vi "Lidar Master V5.2.vi"() -> ()   [LabVIEW 2015]
uses:
  Controls/FPGA Nain State.ctl
  <vilib>/Platform/TimedLoop/XDataNode/timing_clust.ctl
  <vilib>/Platform/TimedLoop/XDataNode/nitl_modes.ctl
  <vilib>/Platform/TimedLoop/XDataNode/wakeup.ctl
  <vilib>/rvi/Emulation/niFpgaGetClockAttributes.vi
  <vilib>/rvi/Emulation/niFpgaSctlEmulationGetInTimedLoop.vi
  <vilib>/rvi/Emulation/niFpgaEmulationReportErrorSimple.vi
  <vilib>/rvi/eio/common/nirviEmuTemplateMethod_errors.vi
  <vilib>/rvi/Emulation/niFpgaCriticalErrorInLSC.vi
  <vilib>/rvi/Emulation/niFpgaProcessEmulError.vi
  <vilib>/rvi/Memory/Memory_Emulation/nirvimemoryFastEmulation.vi
  <vilib>/rvi/Memory/Memory_Emulation/nirvimemoryEmulation.vi
  <vilib>/rvi/Emulation/niFpgaEmulationIsFPGAContextNoSignature.vi
  <vilib>/rvi/DataTransferAndStorage/Container/Common/niFpgaContainerGetUniqueNameForEmu.vi
  <vilib>/rvi/errors/nirviReportUnexpectedCaseInternalError (U32).vi
  <vilib>/rvi/errors/niFpgaSetErrorForExecOnDevCompSimple.vi
  <vilib>/rvi/eio/common/nirviEmuReportErrorAndStop.vi
  <vilib>/rvi/FIFO/Fifo_Resource/nirvififoEmulationSetSize.vi
  <vilib>/rvi/FIFO/Fifo_Resource/nirviFifoEmulationQueueMgr.vi
  <instcachedir>/0/nirviFifoEmulationQueueMgr_E5CAEC123FF24DC58D834DCA3CDAA9B5.lvgen/nirviFifoEmulationQueueMgr_E5CAEC123FF24DC58D834DCA3CDAA9B5_002.vi
  <vilib>/Utility/error.llb/Clear Errors.vi
  <vilib>/rvi/FIFO/Fifo_Resource/nirvififoEmulationCreateLock.vi
  <vilib>/rvi/FIFO/Fifo_Resource/nirvififoEmulationObtainLock.vi
  <vilib>/rvi/FIFO/Fifo_Resource/nirvififoEmulationReleaseLock.vi
  <vilib>/rvi/occurrence/nirviWaitOnOccurrenceBase.vi
  <vilib>/rvi/errors/nirviReportUnexpectedCaseInternalError.vi
  <vilib>/eio/EIONode/EIONode.xnode
  <vilib>/Platform/TimedLoop/XDataNode/XDataNode.xnode
  <vilib>/rvi/DataTransferAndStorage/Container/XNode/niFpgaContainer.xnode
  <vilib>/rvi/FIFO/Fifo_Resource/nirvififoEmulationRead.vi
  <vilib>/eio/EIOMethodNode/EIOMethodNode.xnode
  <vilib>/Platform/TimedLoop/XDataNode/XDNodeRunTimeDep.lvlib
  LIDAR V2 Globals.vi
panel:
  in  "VgaStart":u8
  in  "User Command Commit":bool
  in  "User Command":u8
  in  "User Data 1":u8
  in  "User Data 0":u8
  in  "StartSyncLoop":bool
  out "Trig1":bool
  in  "SendDebugVal":bool
  in  "WriteSenseData":i16
  in  "WriteSensAdd":i16
  in  "WriteSensDataEn":bool
  in  "ActiveSensDeb":u8
  in  "SensScanDeb":bool
  in  "SensorMap":u8[](array[numeric])=[0, 0, 0, 0, 0, 0, 0, 0, 0, 0, 0, 0, 1, 1, 1, 1, 1, 1, 1, 1, 1, 1, 1, 1, 0, 0, 0, 0, 0, 0, 0, 0, 0, 0, 0, 0, 1, 1, 1, 1, 1, 1, 1, 1, 1, 1, 1, 1, 2, 2, 2, 2, 2, 2, 2, 2, 2, 2, 2, 2, 3, 3, 3, 3, 3, 3, 3, 3, 3, 3, 3, 3, 2, 2, 2, 2, 2, 2, 2, 2, 2, 2, 2, 2, 3, 3, 3, 3, 3, 3, 3, 3, 3, 3, 3, 3]
  in  "AiNoOfSamples":u16=99
  out "User Command Idle":bool
  out "User Command Status":u8
  out "User Error":bool
  out "Configured?":bool
  out "PLL Locked":bool
  in  "SendAiCMD":u16
  in  "NoOfSamples":u16=1247
  in  "DOActivate":u16=10
  in  "PulseEnd":u16=25
  in  "VgaAdd":u32
  in  "VgaData":i16
  in  "FillVga":bool
  in  "PowerBit0":bool
  in  "PowerBit1":bool
  in  "ActiveLedIndexDeb":u16
  in  "LedScanDebEn":bool
  out "Port0":u8=2 format="%.0b"
  out "Port1Bit4":bool
  out "Port1Bit5":bool
  out "Port1":u8 format="%.0b"
  in  "ScanMode":bool
  out "PulseIndex":i16=88
  in  "StartAcq":u16=26
  in  "StartPulse":u16=20
  in  "StartES":u16=15
  in  "StopES":u16=30
  out "EnableSignal":bool
  out "ActiveLedIndex":u16=2
  in  "EndOfPulseGen":bool=TRUE
  in  "SamplingEnable":bool
  in  "SingleFrame":bool
  out "MainState":T1=enum."ActivatePulseCycle"
  in  "NoOfLeds":u16=95
  in  "PulsePerLed":i16=199
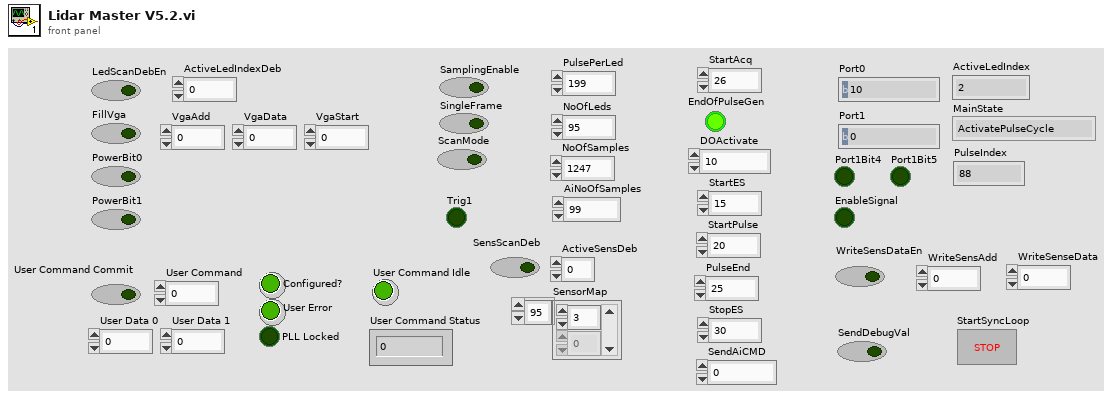
[diagram p1: front panel]
types:
  T1 = typedef "FPGA Nain State.ctl" = enum16{"WaitForStart", "SelectActiveLed", "WaitForNextPulse", "ActivatePulseCycle", "Error"}
  T2 = typedef "XDNodeRunTimeDep.lvlib/timing_clust.ctl" = cluster{"Expected End [f-1]":u64, "Actual End [f-1]":u64, "Finished Late? [f-1]":bool, "Expected End [i-1]":u64, "Actual End [i-1]":u64, "Finished Late? [i-1]":bool, "Expected Start [i]":u64, "Actual Start [i]":u64, "Expected Start [f]":u64, "Actual Start [f]":u64, "Source Name":string, "Structure Name":string, "Period":i64, "Deadline":i64, "Offset":i64, "Start":i64, "Priority":i32, "Timeout":i32, "Mode":T3, "Wakeup Reason":T4, "Error":errorcluster, "Source Type":string, "Secondary Source Type":string, "Global End Time":u64, "Global Start Time":u64, "Frame Duration":u64, "Iteration Duration":u64, "Assigned CPU":i32, "I/O Scan Engine Mode":u32}
  T3 = typedef "XDNodeRunTimeDep.lvlib/nitl_modes.ctl" = enum32{"No Change", "Process missed periods, maintain original phase", "Discard missed periods, maintain original phase", "Process missed periods, ignore original phase", "Discard missed periods, ignore original phase"}
  T4 = typedef "XDNodeRunTimeDep.lvlib/wakeup.ctl" = enum32{"Normal", "Aborted", "Asynchronous wakeup", "Timing source error", "Timed loop error", "Timeout"}
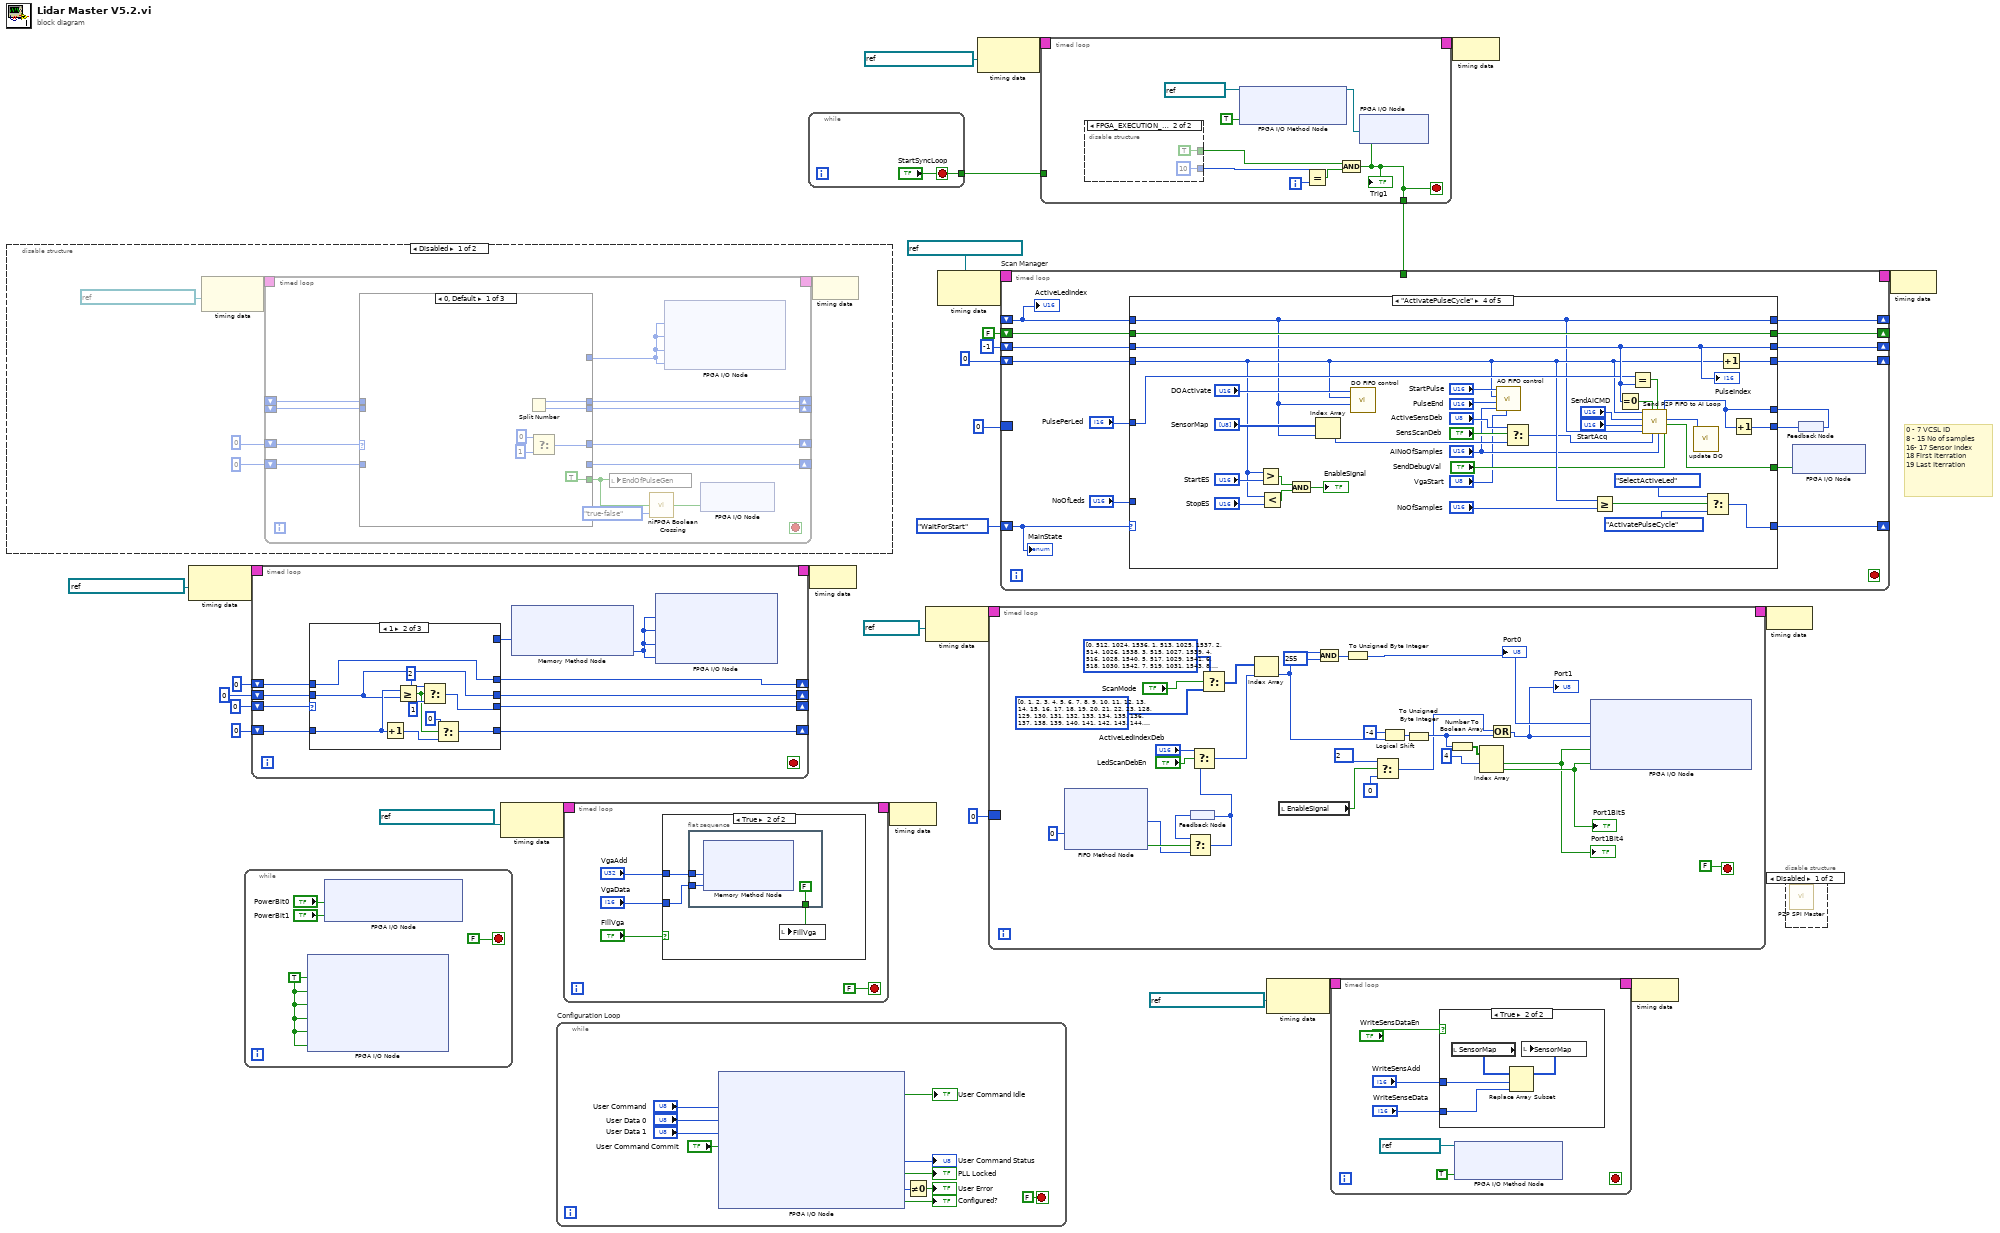
[diagram p0: block diagram]
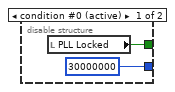
[diagram p3: hidden frame]
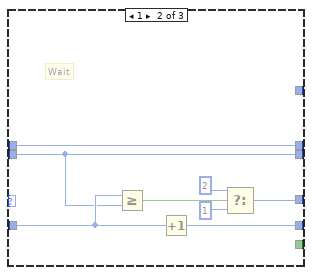
[diagram p5: hidden frame]
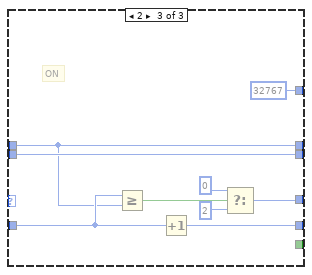
[diagram p6: hidden frame]
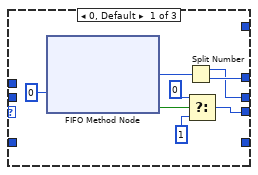
[diagram p8: hidden frame]
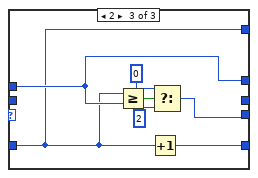
[diagram p9: hidden frame]
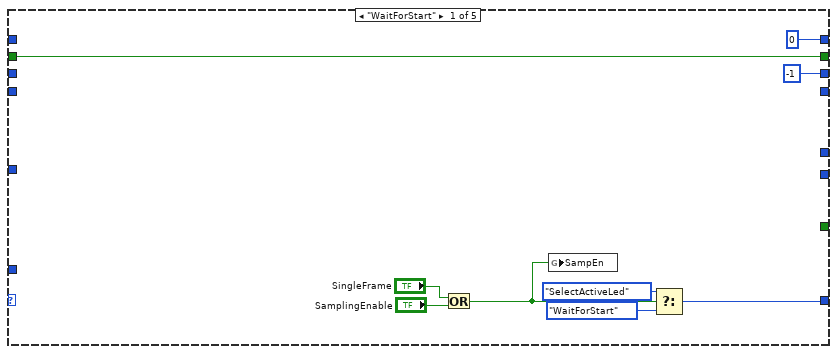
[diagram p11: hidden frame]
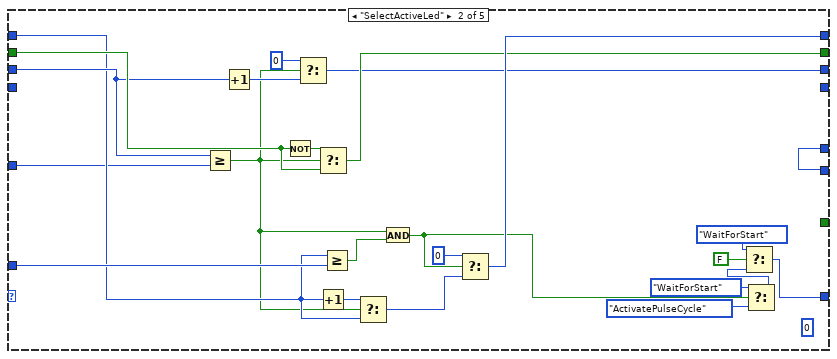
[diagram p12: hidden frame]
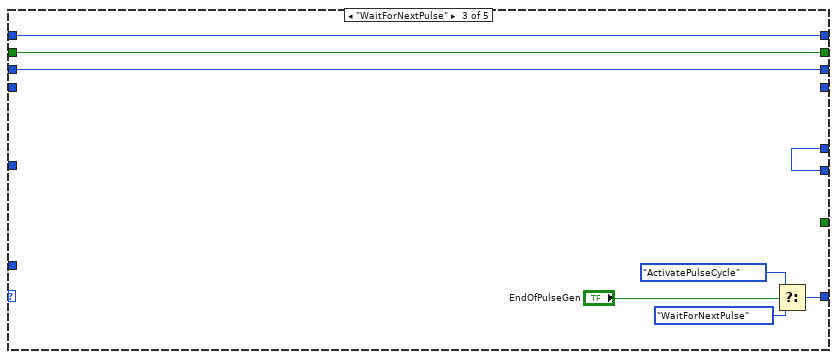
[diagram p13: hidden frame]
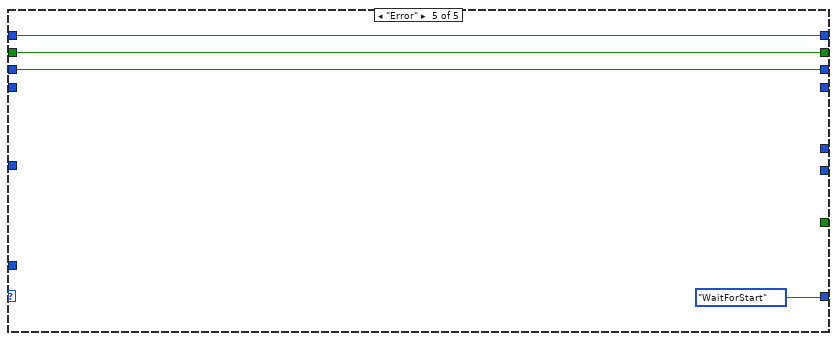
[diagram p14: hidden frame]
diagram:
  # "0 - 7 VCSL ID\n8 - 15 No of samples\n16- 17 Sensor index\n18 First Iterration\n19 Last Iterration"
  n1 = disable-structure shown="Disabled" {
    frame Disabled {
      n2 = node-c288(refnum<k21> "IO Module\\Data Clock" ("Source Name")) -> (w35:T2)
      n3 = timed-loop {
        timing: w35 -> [_]
        timing-out: [_] -> w34
        shift-right: [w46] -> _
        shift-left: i16 0 -> [w47]
        shift-right: [w45] -> _
        shift-left: u32 0 -> [w39]
        shift-right: [w44] -> _
        shift-left: _ -> [w42]
        shift-right: [w43] -> _
        shift-left: _ -> [w41]
        stop <- _ stop-if-true
        n4 = case shown="0, Default" w47 {
          tunnel: [w52 w60 w69] -> w46
          tunnel: [_ w62 w71] -> w45
          tunnel: w39 -> [_ w61 w70]
          tunnel: [w50 w58 w67] -> w44
          tunnel: [w49 w55 w64] -> w43
          tunnel: w42 -> [_ w58 w67]
          tunnel: w41 -> [_ w55 w64]
          tunnel: [_ _ i16 32767 ("IO Module\\AO 0 N")] -> w40
          tunnel: [TRUE _ _] -> w38
          frame 0, Default {
            n5 = Split Number() -> (hi(x)=w49:u16, lo(x)=w50:u16)  [unwired: 1 in]
            n6 = Select(t=i16 0, f=i16 1) -> (s=w54:bool, s? t:f=w52:i16)
          }
          frame 1 {
            # "Wait"
            n7 = Greater Or Equal?(x=w61, y=w58) -> (x >= y?=w59:bool)
            n8 = Increment(x=w61) -> (x+1=w62:u32)
            n9 = Select(t=i16 2, s=w59, f=i16 1) -> (s? t:f=w60:i16)
          }
          frame 2 {
            # "ON"
            n10 = Greater Or Equal?(x=w70, y=w64) -> (x >= y?=w68:bool)
            n11 = Increment(x=w70) -> (x+1=w71:u32)
            n12 = Select(t=i16 0, s=w68, f=i16 2) -> (s? t:f=w69:i16)
          }
        }
        n13 = local write "EndOfPulseGen"(w38) -> ()
        n14 = call <vilib>:"niFPGA Boolean Crossing.vi"("input"=w38, "direction"=enum8{"either", "false-true", "true-false"}."true-false") -> ("crossing"=w36:bool)  [unwired: 7 in]
        n15 = xnode "FPGA I/O Node"("IO Module\\AO 0 N-3"=w40, "IO Module\\AO 0 N-2"=w40, "IO Module\\AO 0 N-1"=w40, "IO Module\\AO 0 N"=w40) -> ()  [unwired: 4 in, 4 out]
        n16 = xnode "FPGA I/O Node"("PXI_Trig0"=w36) -> ()  [unwired: 1 in, 1 out]
      }
      n17 = node-c288(w34) -> ()
    }
    frame Enabled {
    }
  }
  n18 = node-c288(refnum<k21> "IO Module\\Data Clock" ("Source Name")) -> (w17:T2)
  n19 = while {
    stop <- FALSE stop-if-true
    w78 = TRUE ("IO Module\\PFI 0 WE")
    n20 = xnode "FPGA I/O Node"("IO Module\\PFI 0 WE"=w78, "IO Module\\PFI 1 WE"=w78, "IO Module\\PFI 2 WE"=w78, "IO Module\\PFI 3 WE"=w78, "IO Module\\DIO Port 0 WE"=w78, "IO Module\\DIO Port 1 WE"=w78) -> ()  [unwired: 6 in, 6 out]
    n21 = xnode "FPGA I/O Node"("IO Module\\PFI 2 Wr Data"="PowerBit0", "IO Module\\PFI 3 Wr Data"="PowerBit1") -> ()  [unwired: 2 in, 2 out]
  }
  n22 = timed-loop {
    timing: w17 -> [_]
    timing-out: [_] -> w16
    shift-right: [w88] -> _
    shift-left: u16 0 -> [w87]
    shift-right: [w89] -> _
    shift-left: u8 0 -> [w90]
    shift-right: [w86] -> _
    shift-left: u16 0 ("Element") -> [w85]
    shift-right: [w84] -> _
    shift-left: u8 0 -> [w83]
    stop <- _ stop-if-true
    n23 = case shown="1" w90 {
      tunnel: [w95 w104 w112] -> w89
      tunnel: w87 -> [_ w109 w110]
      tunnel: [_ w102 w116] -> w88
      tunnel: w85 -> [_ w106 w111]
      tunnel: [w93 w106 w111] -> w86
      tunnel: [w92 w105 _] -> w84
      tunnel: w83 -> [_ w105 _]
      tunnel: [_ _ w110] -> w82
      frame 0, Default {
        n24 = xnode ("FIFO Method Node")("Timeout"=0) -> ("Element"=w94:u16, "Timed Out?"=w98:bool)  [unwired: 1 in, 1 out]
        n25 = Split Number(x=w94) -> (hi(x)=w92:u8, lo(x)=w93:u8)
        n26 = Select(t=u8 0, s=w98, f=u8 1) -> (s? t:f=w95:u8)
      }
      frame 1 {
        n27 = Increment(x=w109) -> (x+1=w103:u16)
        n28 = Greater Or Equal?(x=w109, y=w105) -> (x >= y?=w100:bool)
        n29 = Select(t=u8 2, s=w100, f=u8 1) -> (s? t:f=w104:u8)
        n30 = Select(t=u16 0, s=w100, f=w103) -> (s? t:f=w102:u16)
      }
      frame 2 {
        n31 = Greater Or Equal?(x=w110, y=w111) -> (x >= y?=w115:bool)
        n32 = Increment(x=w110) -> (x+1=w116:u16)
        n33 = Select(t=u8 0, s=w115, f=u8 2) -> (s? t:f=w112:u8)
      }
    }
    n34 = xnode ("Memory Method Node")("Address"=w82) -> ("Data"=w91:i16)  [unwired: 1 in, 1 out]
    n35 = xnode "FPGA I/O Node"("IO Module\\AO 1 N-3"=w91, "IO Module\\AO 1 N-2"=w91, "IO Module\\AO 1 N-1"=w91, "IO Module\\AO 1 N"=w91) -> ()  [unwired: 4 in, 4 out]
  }
  n36 = node-c288(refnum<k21> "IO Module\\Data Clock" ("Source Name")) -> (w21:T2)
  n37 = while "Configuration Loop" {
    stop <- FALSE stop-if-true
    n38 = xnode "FPGA I/O Node"("IO Module\\User Command"="User Command", "IO Module\\User Data 0"="User Data 0", "IO Module\\User Data 1"="User Data 1", "IO Module\\User Command Commit"="User Command Commit") -> ("IO Module\\User Command Idle"=→"User Command Idle":bool, "IO Module\\User Command Status"=→"User Command Status":u8, "IO Module\\PLL Locked"=→"PLL Locked":bool, "IO Module\\User Error"=w126:u8, "IO Module\\Initialization Done"=→"Configured?":bool)  [unwired: 9 in, 9 out]
    n39 = Not Equal To 0?(x=w126) -> (x != 0?=→"User Error":bool)
  }
  n40 = timed-loop {
    timing: w21 -> [_]
    timing-out: [_] -> w20
    stop <- FALSE stop-if-true
    n41 = case shown="True" "FillVga" {
      tunnel: "VgaAdd" -> [_ w136]
      tunnel: "VgaData" -> [_ w135]
      frame False {
      }
      frame True {
        n42 = flat-sequence {
          tunnel: w136 -> [w139]
          tunnel: w135 -> [w138]
          tunnel: [FALSE ("FillVga")] -> w134
          frame #0 {
            n43 = xnode ("Memory Method Node")("Address"=w139, "Data"=w138) -> ()  [unwired: 1 in, 1 out]
          }
        }
        n44 = local write "FillVga"(w134) -> ()
      }
    }
  }
  n45 = while {
    tunnel: ["StartSyncLoop"] -> w2
    stop <- "StartSyncLoop" stop-if-true
  }
  n46 = node-c288(w16) -> ()
  n47 = node-c288(w20) -> ()
  n48 = node-c288(refnum<k21> "130MHz" ("Source Name")) -> (w28:T2)
  n49 = node-c288(refnum<k21> "IO Module\\Data Clock" ("Source Name")) -> (w30:T2)
  n50 = node-c288(refnum<k21> "PXI Clk10 MHz Clock" ("Source Name")) -> (w6:T2)
  n51 = timed-loop {
    timing: w28 -> [_]
    timing-out: [_] -> w27
    border: u16 0 ("Element") -> [_]
    stop <- FALSE stop-if-true
    n52 = xnode ("FIFO Method Node")("Timeout"=0) -> ("Element"=w151:u16, "Timed Out?"=w152:bool)  [unwired: 1 in, 1 out]
    n53 = feedback #1() -> (w149:u16)
    n54 = Select(t=w149, s=w152, f=w151) -> (s? t:f=w150:u16)
    n55 = feedback-in #1(w150) -> ()
    n56 = Select(t="ActiveLedIndexDeb", s="LedScanDebEn", f=w150) -> (s? t:f=w160:u16)
    n57 = Select(t=u16[] [0, 512, 1024, 1536, 1, 513, 1025, 1537, 2, 514, 1026, 1538, 3, 515, 1027, 1539, 4, 516, 1028, 1540, 5, 517, 1029, 1541, 6, 518, 1030, 1542, 7, 519, 1031, 1543, 8, 520, 1032, 1544, 9, 521, 1033, 1545, 10, 522, 1034, 1546, 11, 523, 1035, 1547, 12, 524, 1036, 1548, 13, 525, 1037, 1549, 14, 526, 1038, 1550, 15, 527, 1039, 1551, 16, 528, 1040, 1552, 17, 529, 1041, 1553, 18, 530, 1042, 1554, 19, 531, 1043, 1555, 20, 532, 1044, 1556, 21, 533, 1045, 1557, 22, 534, 1046, 1558, 23, 535, 1047, 1559, 0, 0, 0, 0, 0, 0, 0, 0, 0, 0, 0, 0, 0, 0, 0, 0, 0, 0, 0, 0, 0, 0, 0, 0, 0, 0, 0, 0, 0, 0, 0, 0, 0, 0, 0, 0, 0, 0, 0, 0, 0, 0, 0, 0, 0, 0, 0, 0, 0, 0, 0, 0, 0, 0, 0, 0, 0, 0, 0, 0, 0, 0, 0, 0, 0, 0, 0, 0, 0, 0, 0, 0, 0, 0, 0, 0, 0, 0, 0, 0, 0, 0, 0, 0, 0, 0, 0, 0, 0, 0, 0, 0, 0, 0, 0, 0, 0, 0, 0, 0, 0, 0, 0, 0, 0, 0, 0, 0, 0, 0, 0, 0, 0, 0, 0, 0, 0, 0, 0, 0, 0, 0, 0, 0, 0, 0, 0, 0, 0, 0, 0, 0, 0, 0, 0, 0, 0, 0, 0, 0, 0, 0, 0, 0, 0, 0, 0, 0, 0, 0, 0, 0, 0, 0, 0, 0, 0, 0, 0, 0, 0, 0, 0, 0, 0, 0, 0, 0, 0, 0, 0, 0, 0, 0, 0, 0, 0, 0, 0, 0, 0, 0, 0, 0, 0, 0, 0, 0, 0, 0, 0, 0, 0, 0, 0, 0, 0, 0, 0, 0, 0, 0, 0, 0, 0, 0, 0, 0, 0, 0, 0, 0, 0, 0, 0, 0, 0, 0, 0, 0, 0, 0, 0, 0] ("Array"), s="ScanMode", f=u16[] [0, 1, 2, 3, 4, 5, 6, 7, 8, 9, 10, 11, 12, 13, 14, 15, 16, 17, 18, 19, 20, 21, 22, 23, 128, 129, 130, 131, 132, 133, 134, 135, 136, 137, 138, 139, 140, 141, 142, 143, 144, 145, 146, 147, 148, 149, 150, 151, 256, 257, 258, 259, 260, 261, 262, 263, 264, 265, 266, 267, 268, 269, 270, 271, 272, 273, 274, 275, 276, 277, 278, 279, 384, 385, 386, 387, 388, 389, 390, 391, 392, 393, 394, 395, 396, 397, 398, 399, 400, 401, 402, 403, 404, 405, 406, 407, 0, 0, 0, 0, 0, 0, 0, 0, 0, 0, 0, 0, 0, 0, 0, 0, 0, 0, 0, 0, 0, 0, 0, 0, 0, 0, 0, 0, 0, 0, 0, 0, 0, 0, 0, 0, 0, 0, 0, 0, 0, 0, 0, 0, 0, 0, 0, 0, 0, 0, 0, 0, 0, 0, 0, 0, 0, 0, 0, 0, 0, 0, 0, 0, 0, 0, 0, 0, 0, 0, 0, 0, 0, 0, 0, 0, 0, 0, 0, 0, 0, 0, 0, 0, 0, 0, 0, 0, 0, 0, 0, 0, 0, 0, 0, 0, 0, 0, 0, 0, 0, 0, 0, 0, 0, 0, 0, 0, 0, 0, 0, 0, 0, 0, 0, 0, 0, 0, 0, 0, 0, 0, 0, 0, 0, 0, 0, 0, 0, 0, 0, 0, 0, 0, 0, 0, 0, 0, 0, 0, 0, 0, 0, 0, 0, 0, 0, 0, 0, 0, 0, 0, 0, 0, 0, 0, 0, 0, 0, 0, 0, 0, 0, 0, 0, 0, 0, 0, 0, 0, 0, 0, 0, 0, 0, 0, 0, 0, 0, 0, 0, 0, 0, 0, 0, 0, 0, 0, 0, 0, 0, 0, 0, 0, 0, 0, 0, 0, 0, 0, 0, 0, 0, 0, 0, 0, 0, 0, 0, 0, 0, 0, 0, 0, 0, 0, 0, 0, 0, 0, 0, 0, 0, 0] ("Array")) -> (s? t:f=w155:u16[])
    n58 = Index Array(array=w155, index=w160) -> (element=w145:u16)
    n59 = local read "EnableSignal"() -> (w153:bool)
    n60 = And(x=w145, y=u16 255) -> (x .and. y?=w165:u16)
    n61 = To Unsigned Byte Integer(number=w165) -> (unsigned 8bit integer=w163:u8)
    "Port0" <- w163
    n62 = Select(t=u8 2, s=w153, f=u8 0) -> (s? t:f=w144:u8)
    n63 = Logical Shift(y=i16 -4, x=w145) -> (x << y=w164:u16)
    n64 = To Unsigned Byte Integer(number=w164) -> (unsigned 8bit integer=w162:u8)
    n65 = Number To Boolean Array(number=w162) -> (Boolean array=w169:bool[])
    n66 = Index Array(array=w169, index #1=4 ("index")) -> (element #1=w147:bool, element #2=w148:bool)  [unwired: 1 in]
    "Port1Bit4" <- w147
    "Port1Bit5" <- w148
    n67 = Or(x=w144, y=w162) -> (x .or. y?=w161:u8)
    "Port1" <- w161
    n68 = xnode "FPGA I/O Node"("IO Module\\DIO Port 0 Wr Data"=w163, "IO Module\\DIO Port 1 Wr Data"=w161, "IO Module\\PFI 0 Wr Data"=w147, "IO Module\\PFI 1 Wr Data"=w148) -> ()  [unwired: 4 in, 4 out]
  }
  n69 = timed-loop {
    timing: w6 -> [_]
    timing-out: [_] -> w5
    tunnel: [w178] -> w3
    tunnel: w2 -> [_]
    i -> [w181]
    stop <- w178 stop-if-true
    n70 = disable-structure shown="FPGA_EXECUTION_MODE==DEV_COMPUTER_SIM_IO" {
      disable-tunnel: [w183 TRUE ("PLL Locked")] -> w179
      disable-tunnel: [30000000 ("x") 10 ("x")] -> w174
      frame condition #0 (active) {
        n71 = local read "PLL Locked"() -> (w183:bool)
      }
      frame condition #1 {
      }
    }
    n72 = xnode "FPGA I/O Method Node"("FPGA I/O In"=refnum<k21> "PXI_Trig1", "Enable"=TRUE) -> ("FPGA I/O Out"=w175:refnum<k21>)
    n73 = Equal?(x=w174, y=w181) -> (x = y?=w180:bool)
    n74 = And(x=w179, y=w180) -> (x .and. y?=w178:bool)
    "Trig1" <- w178
    n75 = xnode "FPGA I/O Node"("I/O Item"=w178, "FPGA I/O In"=w175) -> ()  [unwired: 1 out]
  }
  n76 = timed-loop "Scan Manager" {
    timing: w30 -> [_]
    timing-out: [_] -> w29
    shift-right: [w201] -> _
    shift-left: FPGA_Nain_State."WaitForStart" ("MainState") -> [w202]
    shift-right: [w196] -> _
    shift-left: _ -> [w191]
    shift-right: [w198] -> _
    shift-left: FALSE -> [w200]
    shift-right: [w199] -> _
    shift-left: i16 -1 -> [w197]
    shift-right: [w192] -> _
    shift-left: u16 0 -> [w193]
    border: u32 0 -> [_]
    tunnel: w3 -> [_]
    stop <- _ stop-if-true
    n77 = feedback #2() -> (w188:u32)
    n78 = case shown="\"ActivatePulseCycle\"" w202 {
      tunnel: [w209 w232 w239 w275 FPGA_Nain_State."WaitForStart" ("MainState")] -> w201
      tunnel: [u16 0 ("ActiveLedIndex") w228 w238 w254 w282] -> w196
      tunnel: w191 -> [_ w220 w238 w254 w282]
      tunnel: [w206 w227 w243 w274 w281] -> w198
      tunnel: w200 -> [w206 w230 w243 w274 w281]
      tunnel: [i16 -1 ("t") w223 w242 w259 w280] -> w199
      tunnel: w197 -> [_ w226 w242 w259 w280]
      tunnel: "NoOfLeds" -> [_ w222 _ _ _]
      tunnel: "PulsePerLed" -> [_ w213 _ w258 _]
      tunnel: w193 -> [_ _ _ w255 _]
      tunnel: [_ _ _ w273 _] -> w192
      tunnel: [_ _ _ w250 _] -> w190
      tunnel: w188 -> [_ w212 w236 w248 _]
      tunnel: [_ w212 w236 w249 _] -> w189
      frame "WaitForStart" {
        n79 = Or(x="SingleFrame", y="SamplingEnable") -> (x .or. y?=w203:bool)
        n80 = global write "LIDAR V2 Globals.vi" "SampEn"(w203) -> ()
        n81 = Select(t=FPGA_Nain_State."SelectActiveLed" ("MainState"), s=w203, f=FPGA_Nain_State."WaitForStart" ("MainState")) -> (s? t:f=w209:T1)
      }
      frame "SelectActiveLed" {
        (unwired) u8 0
        n82 = Greater Or Equal?(x=w226, y=w213) -> (x >= y?=w215:bool)
        n83 = Increment(x=w226) -> (x+1=w225:i16)
        n84 = Not(x=w230) -> (.not. x?=w229:bool)
        n85 = Select(t=i16 0, s=w215, f=w225) -> (s? t:f=w223:i16)
        n86 = Select(t=w229, s=w215, f=w230) -> (s? t:f=w227:bool)
        n87 = Increment(x=w220) -> (x+1=w218:u16)
        n88 = Greater Or Equal?(x=w220, y=w222) -> (x >= y?=w216:bool)
        n89 = Select(t=w218, s=w215, f=w220) -> (s? t:f=w219:u16)
        n90 = And(x=w215, y=w216) -> (x .and. y?=w214:bool)
        n91 = Select(t=u16 0, s=w214, f=w219) -> (s? t:f=w228:u16)
        n92 = Select(t=FPGA_Nain_State."WaitForStart" ("MainState"), s=w214, f=FPGA_Nain_State."ActivatePulseCycle" ("MainState")) -> (s? t:f=w233:T1)
        n93 = Select(t=FPGA_Nain_State."WaitForStart" ("MainState"), s=FALSE, f=w233) -> (s? t:f=w232:T1)
      }
      frame "WaitForNextPulse" {
        n94 = Select(t=FPGA_Nain_State."ActivatePulseCycle" ("MainState"), s="EndOfPulseGen", f=FPGA_Nain_State."WaitForNextPulse" ("MainState")) -> (s? t:f=w239:T1)
      }
      frame "ActivatePulseCycle" {
        n95 = Greater?(x=w255, y="StartES") -> (0:w268:bool)
        n96 = Less?(x=w255, y="StopES") -> (x < y?=w269:bool)
        n97 = And(x=w268, y=w269) -> (x .and. y?=→"EnableSignal":bool)
        n98 = Index Array(array="SensorMap", index=w254) -> (element=w253:u8)
        n99 = call "DO FIFO control.vi"("PulseData"=w254, "Counter"=w255, "DOActivate"="DOActivate") -> ()  [unwired: 9 in]
        n100 = call "AO FIFO control.vi"("StartVGA"="VgaStart", "NoOfSamples"="AiNoOfSamples", "PulseEnd"="PulseEnd", "Counter"=w255, "PulseStart"="StartPulse") -> ()  [unwired: 7 in]
        n101 = Select(t="ActiveSensDeb", s="SensScanDeb", f=w253) -> (s? t:f=w252:u8)
        n102 = Greater Or Equal?(x=w255, y="NoOfSamples") -> (x >= y?=w278:bool)
        n103 = Equal To 0?(x=w259) -> (x = 0?=w261:bool)
        n104 = Equal?(x=w258, y=w259) -> (x = y?=w260:bool)
        n105 = call "Send P2P FIFO to AI Loop.vi"("SendDebugVal"="SendDebugVal", "DebugVals"=w248, "NoOfSamples"="AiNoOfSamples", "LastIterration"=w260, "SensorID"=w252, "FirstIterration"=w261, "ActiveLedIndex"=w254, "SendAiTrig"="StartAcq", "SendAiCMD"="SendAiCMD", "TimingCounter"=w255) -> ("Trig"=w250:bool, "DIOControl"=w244:u8)
        n106 = call "update DO.vi"("Control"=w244) -> ()  [unwired: 11 in]
        n107 = Select(t=FPGA_Nain_State."SelectActiveLed" ("MainState"), s=w278, f=FPGA_Nain_State."ActivatePulseCycle" ("MainState")) -> (s? t:f=w275:T1)
        n108 = Increment(x=w255) -> (x+1=w273:u16)
        n109 = Increment(x=w248) -> (x+1=w249:u32)
        "PulseIndex" <- w259
      }
      frame "Error" {
      }
    }
    n110 = xnode "FPGA I/O Node"("PXI_Trig0"=w190) -> ()  [unwired: 1 in, 1 out]
    n111 = feedback-in #2(w189) -> ()
    "MainState" <- w202
    "ActiveLedIndex" <- w191
  }
  n112 = node-c288(refnum<k21> "IO Module\\Data Clock" ("Source Name")) -> (w10:T2)
  n113 = timed-loop {
    timing: w10 -> [_]
    timing-out: [_] -> w9
    stop <- _ stop-if-true
    n114 = case shown="True" "WriteSensDataEn" {
      tunnel: "WriteSensAdd" -> [_ w291]
      tunnel: "WriteSenseData" -> [_ w290]
      frame False {
      }
      frame True {
        n115 = local read "SensorMap"() -> (w293:u8[])
        n116 = Replace Array Subset(array=w293, new element=w290, index=w291) -> (w292:u8[])
        n117 = local write "SensorMap"(w292) -> ()
      }
    }
    n118 = xnode "FPGA I/O Method Node"("FPGA I/O In"=refnum<k21> "PXI_Trig0", "Enable"=TRUE) -> ()  [unwired: 1 out]
  }
  n119 = node-c288(w5) -> ()
  n120 = node-c288(w9) -> ()
  n121 = node-c288(w27) -> ()
  n122 = disable-structure shown="Disabled" {
    frame Disabled {
      n123 = call "P2P SPI Master.vi"() -> ()  [unwired: 12 in]
    }
    frame Enabled {
    }
  }
  n124 = node-c288(w29) -> ()
